vi "crc32.test.vi"() -> ()   [LabVIEW 2020]
uses:
  <vilib>/Platform/TimedLoop/XDataNode/timing_clust.ctl
  <vilib>/Platform/TimedLoop/XDataNode/nitl_modes.ctl
  <vilib>/Platform/TimedLoop/XDataNode/wakeup.ctl
  <vilib>/rvi/Emulation/niFpgaSctlEmulationGetInTimedLoop.vi
  <vilib>/rvi/Emulation/niFpgaEmulationReportErrorSimple.vi
  <vilib>/rvi/Emulation/niFpgaGetClockAttributes.vi
  <vilib>/rvi/Emulation/niFpgaCriticalErrorInLSC.vi
  <vilib>/platform/TimedLoop/XDataNode/XDataNode.xnode
  <vilib>/Platform/TimedLoop/XDataNode/XDNodeRunTimeDep.lvlib
  fpganow.common.fpga.lvlib
panel:
  out "CRC32.out":u32 format="%.0x"
  in  "Data in":u64 format="%.0x"
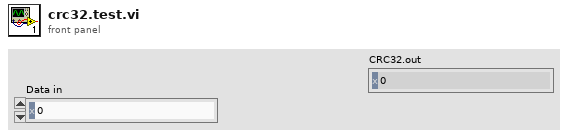
[diagram p1: front panel]
types:
  T1 = typedef "XDNodeRunTimeDep.lvlib/timing_clust.ctl" = cluster{"Expected End [f-1]":u64, "Actual End [f-1]":u64, "Finished Late? [f-1]":bool, "Expected End [i-1]":u64, "Actual End [i-1]":u64, "Finished Late? [i-1]":bool, "Expected Start [i]":u64, "Actual Start [i]":u64, "Expected Start [f]":u64, "Actual Start [f]":u64, "Source Name":string, "Structure Name":string, "Period":i64, "Deadline":i64, "Offset":i64, "Start":i64, "Priority":i32, "Timeout":i32, "Mode":T2, "Wakeup Reason":T3, "Error":errorcluster, "Source Type":string, "Secondary Source Type":string, "Global End Time":u64, "Global Start Time":u64, "Frame Duration":u64, "Iteration Duration":u64, "Assigned CPU":i32, "I/O Scan Engine Mode":u32}
  T2 = typedef "XDNodeRunTimeDep.lvlib/nitl_modes.ctl" = enum32{"No Change", "Process missed periods, maintain original phase", "Discard missed periods, maintain original phase", "Process missed periods, ignore original phase", "Discard missed periods, ignore original phase"}
  T3 = typedef "XDNodeRunTimeDep.lvlib/wakeup.ctl" = enum32{"Normal", "Aborted", "Asynchronous wakeup", "Timing source error", "Timed loop error", "Timeout"}
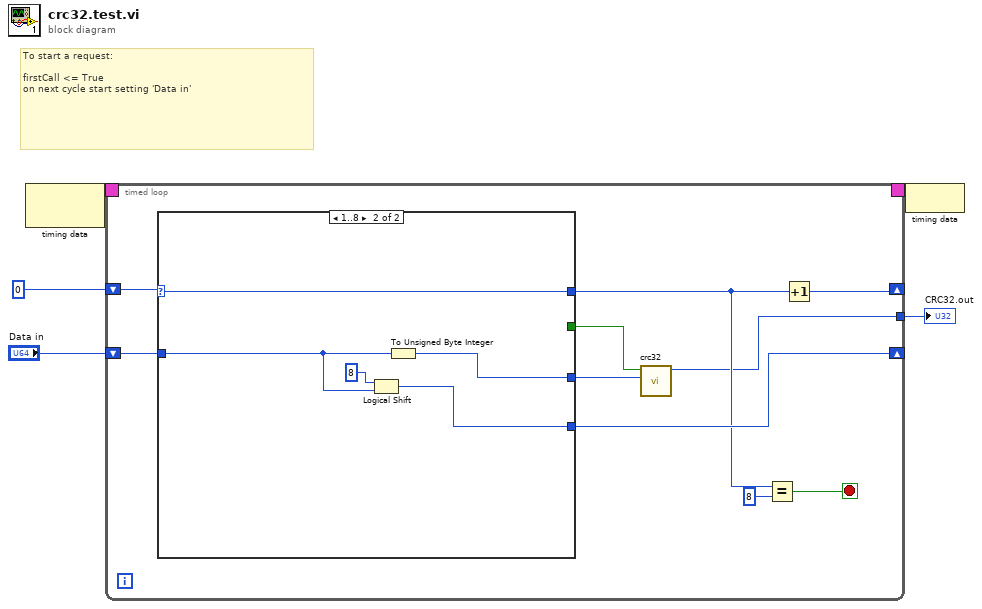
[diagram p0: block diagram]
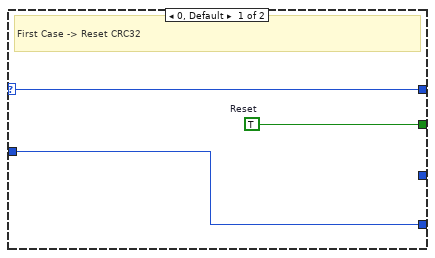
[diagram p2: hidden frame]
diagram:
  # "To start a request:\n\nfirstCall <= True\non next cycle start setting 'Data in'"
  n1 = node-c288() -> (w5:T1)  [unwired: 1 in]
  n2 = timed-loop {
    timing: w5 -> [_]
    timing-out: [_] -> w4
    shift-right: [w10] -> _
    shift-left: "Data in" -> [w13]
    shift-right: [w11] -> _
    shift-left: u8 0 -> [w15]
    tunnel: [w6] -> w1
    stop <- w9 stop-if-true
    n3 = case shown="1..8" w15 {
      selector: w15 -> [w17 w23]
      tunnel: [w18 _] -> w14
      tunnel: w13 -> [w16 w19]
      tunnel: [_ w22] -> w12
      tunnel: [w17 w23] -> w8
      tunnel: [w16 w21] -> w10
      frame 0, Default {
        w18 = TRUE  # Reset
        # "First Case -> Reset CRC32"
      }
      frame 1..8 {
        n4 = Logical Shift(y=u8 8 ("x"), x=w19) -> (x << y=w21:u64)
        n5 = To Unsigned Byte Integer(number=w19) -> (unsigned 8bit integer=w22:u8)
      }
    }
    n6 = call "crc32.vi"("Data.in"=w12, "Reset"=w14) -> ("CRC32.out"=w6:u32)  [unwired: 9 in]
    n7 = Equal?(x=w8, y=u8 8) -> (x = y?=w9:bool)
    n8 = Increment(x=w8) -> (x+1=w11:u8)
  }
  "CRC32.out" <- w1
  n9 = node-c288(w4) -> ()
